vi "Read Step_size.vi"(8 "error in (no error)":errorcluster, 11 "Dynamic-System in":refnum<class "Dynamic-System.lvclass">) -> (0 "error out":errorcluster, 2 "Step_size":dbl, 3 "Dynamic-System out":refnum<class "Dynamic-System.lvclass">)   [LabVIEW 2025, in "Dynamic-System.lvclass"]
uses:
  Dynamic-System.lvclass
  Dynamic-System.lvclass/Dynamic-System.ctl
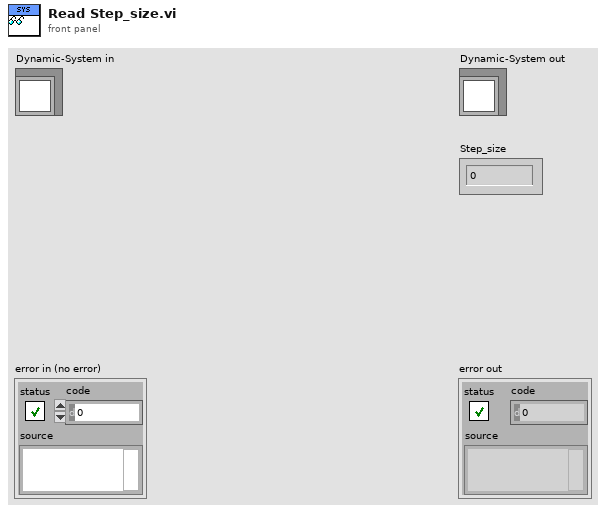
[diagram p1: front panel]
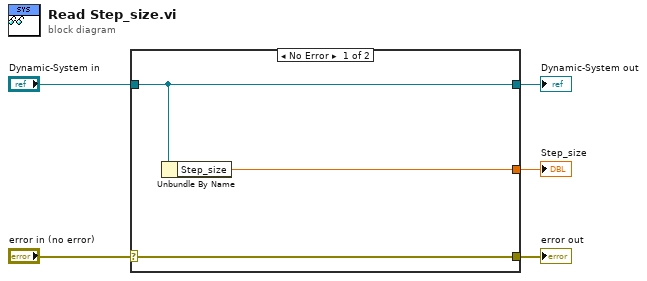
[diagram p0: block diagram]
diagram:
  n1 = case shown="No Error" "error in (no error)" {
    selector: "error in (no error)" -> [w8 w9]
    tunnel: [w8 w9] -> w4
    tunnel: [w7 w10] -> w2
    tunnel: "Dynamic-System in" -> [w7 w10]
    tunnel: [w6 _] -> w1
    frame No Error {
      n2 = Unbundle By Name(w7) -> ("Step_size"=w6:dbl)
    }
    frame Error {
    }
  }
  "error out" <- w4
  "Dynamic-System out" <- w2
  "Step_size" <- w1
